vi "Run.vi"(9 "Team in":refnum<class "Team.lvclass">, 11 "MySquare in":refnum<class "MySquare.lvclass">) -> (1 "Team out":refnum<class "Team.lvclass">, 2 "Run Result":T1, 3 "MySquare out":refnum<class "MySquare.lvclass">)   [LabVIEW 2020, in "Rain.lvlib" / "MySquare.lvclass"]
doc: "This VI is called on every active square each turn of the game for the square to decide what action to take."
uses:
  MySquare.lvclass
  MySquare.lvclass/MySquare.ctl
  MyTeam/MyTeam.lvclass
  SquareBattle/Square/Square.lvclass
  SquareBattle/Action.ctl
  SquareBattle/SquareBattle.lvlib
  SquareBattle/Direction.ctl
  SquareBattle/Run Result.ctl
  C:/dev/sol-squarebattle/SquareBattle/Square/Square.lvclass
  C:/dev/sol-squarebattle/Squares/Rain/SquareTeam/MySquare/MySquare.lvclass
  C:/dev/sol-squarebattle/SquareBattle/Team/Team.lvclass
  C:/dev/sol-squarebattle/Squares/Rain/SquareTeam/MyTeam/MyTeam.lvclass
  SquareBattle/Team/Team.lvclass
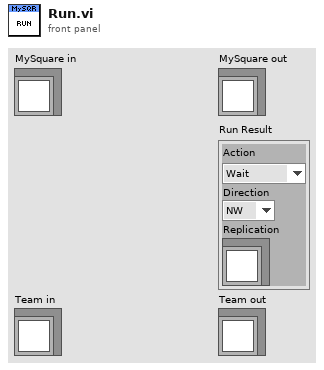
[diagram p1: front panel]
types:
  T1 = typedef "SquareBattle.lvlib/Run Result.ctl" = cluster{"Action":T2, "Direction":T3, "Replication":refnum<class "Square.lvclass">}
  T2 = typedef "SquareBattle.lvlib/Action.ctl" = enum16{"Wait", "Move", "Attack", "Replicate"}
  T3 = typedef "SquareBattle.lvlib/Direction.ctl" = enum16{"NW", "N", "NE", "E", "SE", "S", "SW", "W"}
  T4 = enum16{"NW", "N", "NE", "E", "SE", "S", "SW", "W"}[]
  T5 = typedef "SquareBattle.lvlib/Location Status.ctl" = cluster{"Empty":bool, "Friend":bool, "Enemy":bool}
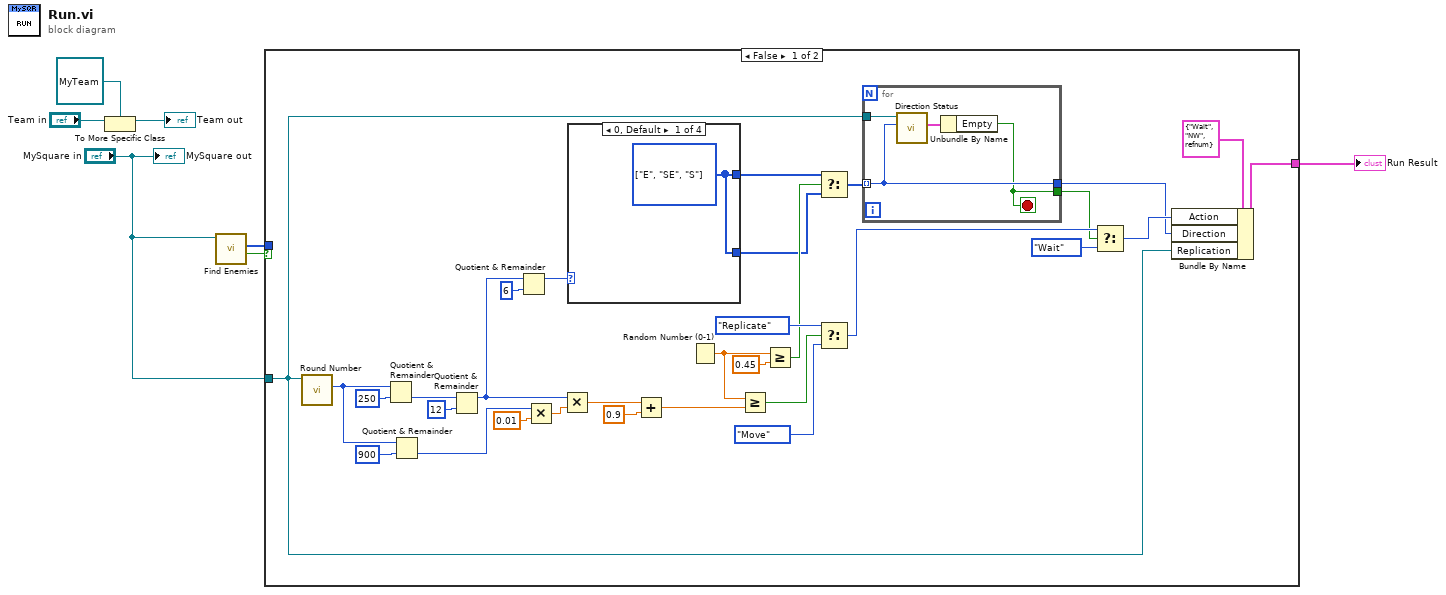
[diagram p0: block diagram]
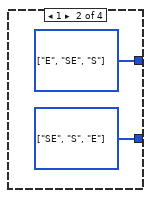
[diagram p2: hidden frame]
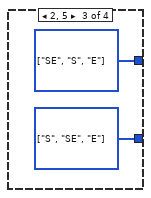
[diagram p3: hidden frame]
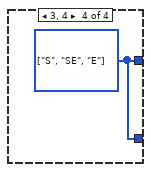
[diagram p4: hidden frame]
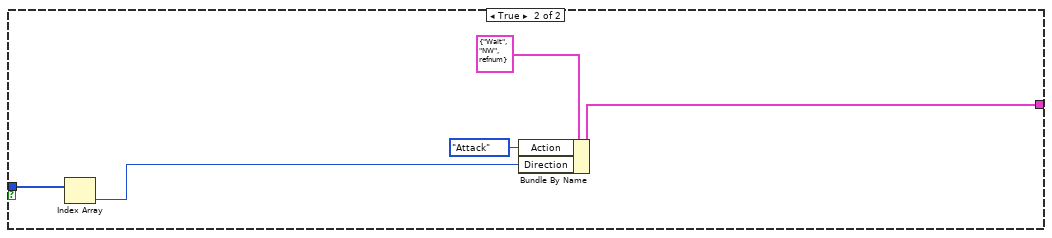
[diagram p5: hidden frame]
diagram:
  n1 = To More Specific Class(target class=refnum<class "MyTeam.lvclass"> refnum ("SquareTeam.lvlib:MyTeam.lvclass"), reference="Team in") -> (specific class reference=→"Team out":refnum<class "MyTeam.lvclass">)  [unwired: 1 in, 1 out]
  n2 = call "Find Enemies.vi"("Square"="MySquare in") -> ("Any Enemies?"=w4:bool, "Enemy Directions"=w2:T3[])  [unwired: 9 in]
  n3 = case shown="False" w4 {
    tunnel: [w11 w52] -> w3
    tunnel: w2 -> [_ w51]
    tunnel: "MySquare in" -> [w9 _]
    frame False {
      n4 = call "Round Number.vi"("Square in"=w9) -> ("Round Number"=w13:u32)  [unwired: 10 in]
      n5 = Quotient & Remainder(x=w13, y=250) -> (floor(x/y)=w25:u32)  [unwired: 1 out]
      n6 = Quotient & Remainder(x=w13, y=900) -> (floor(x/y)=w16:u32)  [unwired: 1 out]
      n7 = Quotient & Remainder(x=w25, y=12) -> (x-y*floor(x/y)=w19:u32)  [unwired: 1 out]
      n8 = Quotient & Remainder(x=w19, y=6) -> (x-y*floor(x/y)=w18:u32)  [unwired: 1 out]
      n9 = Multiply(x=w16, y=0.01) -> (x*y=w14:dbl)
      n10 = Multiply(x=w19, y=w14) -> (x*y=w24:dbl)
      n11 = case shown="0, Default" w18 {
        tunnel: [w39 w41 w43 w44] -> w29
        tunnel: [w39 w40 w42 w44] -> w30
        frame 0, Default {
          w39 = T4 [enum."E", enum."SE", enum."S"] items=["NW", "N", "NE", "E", "SE", "S", "SW", "W"]
        }
        frame 1 {
          w40 = T4 [enum."SE", enum."S", enum."E"] items=["NW", "N", "NE", "E", "SE", "S", "SW", "W"]
          w41 = T4 [enum."E", enum."SE", enum."S"] items=["NW", "N", "NE", "E", "SE", "S", "SW", "W"]
        }
        frame 2, 5 {
          w42 = T4 [enum."S", enum."SE", enum."E"] items=["NW", "N", "NE", "E", "SE", "S", "SW", "W"]
          w43 = T4 [enum."SE", enum."S", enum."E"] items=["NW", "N", "NE", "E", "SE", "S", "SW", "W"]
        }
        frame 3, 4 {
          w44 = T4 [enum."S", enum."SE", enum."E"] items=["NW", "N", "NE", "E", "SE", "S", "SW", "W"]
        }
      }
      n12 = Add(x=w24, y=0.9) -> (x+y=w22:dbl)
      n13 = Random Number (0-1)() -> (number: 0 to 1=w27:dbl)
      n14 = Greater Or Equal?(x=w27, y=w22) -> (x >= y?=w33:bool)
      n15 = Greater Or Equal?(x=w27, y=0.45) -> (x >= y?=w31:bool)
      n16 = Select(t=w29, s=w31, f=w30) -> (s? t:f=w28:T4)
      n17 = Select(t=enum16{"Wait", "Move", "Attack", "Replicate"}."Replicate" ("Action"), s=w33, f=enum16{"Wait", "Move", "Attack", "Replicate"}."Move" ("Action")) -> (s? t:f=w36:enum16{"Wait", "Move", "Attack", "Replicate"})
      n18 = for {
        tunnel: [w45] -> w35
        tunnel: w28 -> [w47] mode=indexing
        tunnel: [w47] -> w8
        tunnel: w9 -> [w48]
        stop <- w45 stop-if-true
        n19 = call "Direction Status.vi"("Direction"=w47, "Square"=w48) -> ("Status"=w46:T5)  [unwired: 9 in]
        n20 = Unbundle By Name(w46) -> ("Empty"=w45:bool)
      }
      n21 = Select(t=w36, s=w35, f=enum16{"Wait", "Move", "Attack", "Replicate"}."Wait" ("Action")) -> (s? t:f=w10:enum16{"Wait", "Move", "Attack", "Replicate"})
      n22 = Bundle By Name(cluster=T1 {"Action"=enum."Wait", "Direction"=enum."NW", "Replication"=refnum} ("Run Result"), "Action"=w10, "Direction"=w8, "Replication"=w9) -> (w11:T1)
    }
    frame True {
      n23 = Index Array(array=w51) -> (element=w50:T3)  [unwired: 1 in]
      n24 = Bundle By Name(cluster=T1 {"Action"=enum."Wait", "Direction"=enum."NW", "Replication"=refnum} ("Run Result"), "Action"=Action."Attack", "Direction"=w50) -> (w52:T1)
    }
  }
  "Run Result" <- w3
  "MySquare out" <- "MySquare in"
